vi "Error Handler - Event Handling Loop.vi"(8 "error in (no error)":errorcluster caption="에러 입력(에러 없음)", 10 "Ignore Errors (Runtime)":i32[](array[numeric]) caption="에러 무시 (런타임)", 11 "Message Queue":refnum<queue> caption="메시지 큐") -> (0 "dup error in":errorcluster caption="에러 입력 복제", 3 "dup Message Queue":refnum<queue> caption="메시지 큐 복제")   [LabVIEW 2018, in "Message Queue.lvlib"]
doc: "이벤트 핸들링 루프에서 발생한 에러를 무시하거나 \"에러\" 메시지를 생성하여 처리합니다."
uses:
  Message Queue.lvlib
  Message Cluster.ctl
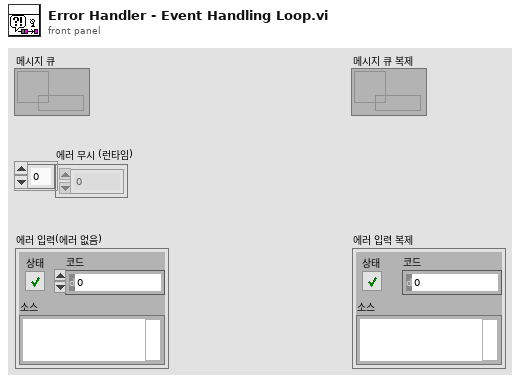
[diagram p1: front panel]
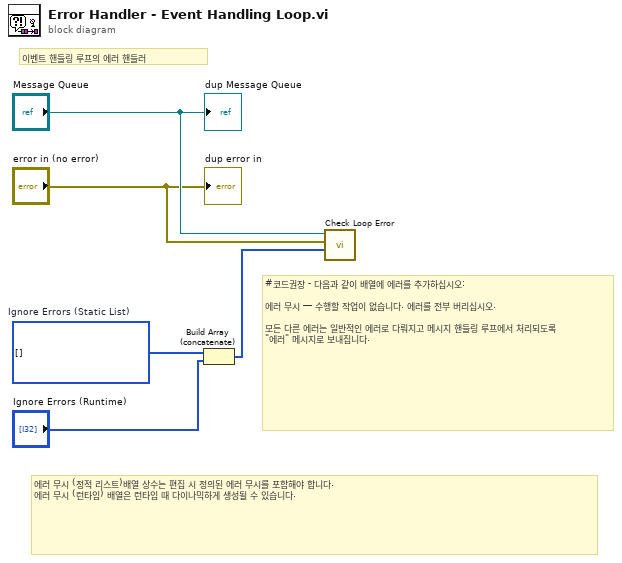
[diagram p0: block diagram]
diagram:
  w3 = i32[] []  # Ignore Errors (Static List)
  # "에러 무시 (정적 리스트)배열 상수는 편집 시 정의된 에러 무시를 포함해야 합니다.\n에러 무시 (런타임) 배열은 런타임 때 다이나믹하게 생성될 수 있습니다."
  # "#코드권장 - 다음과 같이 배열에 에러를 추가하십시오:\n\n에러 무시 ― 수행할 작업이 없습니다. 에러를 전부 버리십시오.\n\n모든 다른 에러는 일반적인 에러로 다뤄지고 메시지 핸들링 루프에서 처리되도록 \"에러\" 메시지로 보내집니다."
  # "이벤트 핸들링 루프의 에러 핸들러"
  n1 = Build Array (concatenate)(w3, "Ignore Errors (Runtime)") -> (w1:i32[])
  n2 = call "Check Loop Error.vi"("Ignore Errors"=w1, "error to process"="error in (no error)", "Message Queue"="Message Queue") -> ()  [unwired: 7 in, 2 out]
  "dup Message Queue" <- "Message Queue"
  "dup error in" <- "error in (no error)"
